vi "convert_int32Array_to_string.vi"(2 "Max Elements Count (All)":i32=-1, 4 "I32 array in":i32[](array[numeric]), 5 "String to add before (\"\")":string) -> (1 "string out":string)   [LabVIEW 2014, in "rszvl_rsidr_core.lvlib"]
uses:
  rszvl_rsidr_core.lvlib
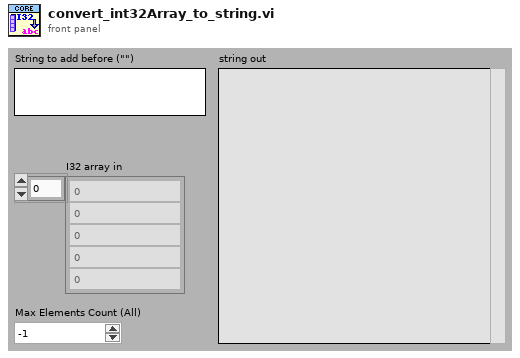
[diagram p1: front panel]
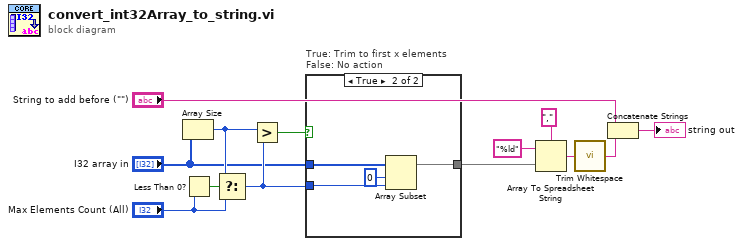
[diagram p0: block diagram]
diagram:
  n1 = Array Size(array="I32 array in") -> (size(s)=w5:i32)
  n2 = Less Than 0?(x="Max Elements Count (All)") -> (x < 0?=w7:bool)
  n3 = Select(t=w5, s=w7, f="Max Elements Count (All)") -> (s? t:f=w3:i32)
  n4 = Greater?(x=w5, y=w3) -> (0:w4:bool)
  n5 = case "True: Trim to first x elements\nFalse: No action" shown="True" w4 {
    tunnel: [w14 w15] -> w1
    tunnel: "I32 array in" -> [w14 w18]
    tunnel: w3 -> [_ w16]
    frame False {
    }
    frame True {
      n6 = Array Subset(array=w18, index=0, length=w16) -> (w15:i32[])
    }
  }
  n7 = Array To Spreadsheet String(delimiter (Tab)=",", array=w1, 3:"%ld" ("format string")) -> (spreadsheet string=w11:string)
  n8 = call "Trim Whitespace.vi"("string"=w11) -> ("trimmed string"=w9:string)  [unwired: 1 in]
  n9 = Concatenate Strings("String to add before (\"\")", w9) -> (→"string out":string)
